vi "StartTrial.vi"(8 "error in (no error)":errorcluster, 11 "TrialBasedExperiment in":refnum<class "OriDiscExperiment.lvclass">) -> (0 "error out":errorcluster, 3 "TrialBasedExperiment out":refnum<class "OriDiscExperiment.lvclass">)   [LabVIEW 2011, in "OriDiscExperiment.lvclass"]
uses:
  OriDiscExperiment.lvclass
  OriDiscExperiment.lvclass/OriDiscExperiment.ctl
  TwoAfcEye/TwoAfcEye.lvclass
panel:
  in  "condRepeatType":string(combo)="None"
  in  "punishType":string(combo)="IncorrRespAndAborts"
  in  "classShown":bool
  in  "classOverride":bool
  in  "correctTargetOnly":bool
  in  "cueTime":dbl
  in  "punishTime":dbl
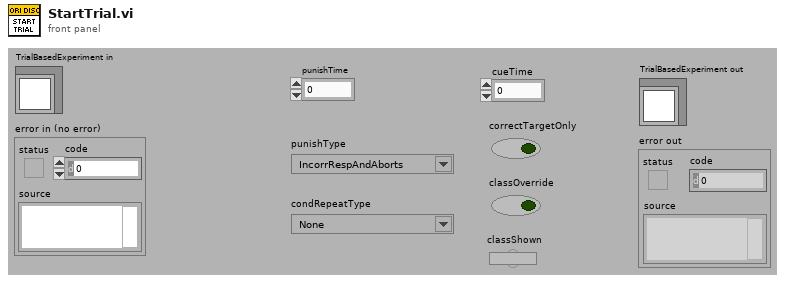
[diagram p1: front panel]
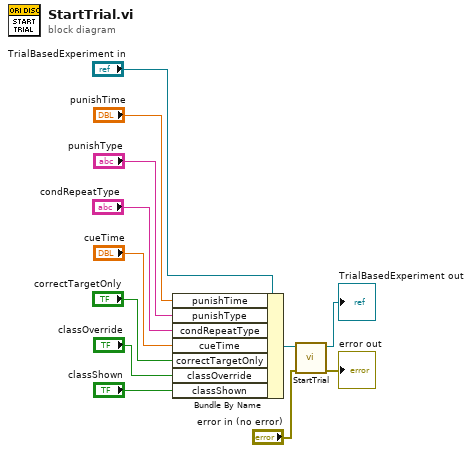
[diagram p0: block diagram]
diagram:
  n1 = Bundle By Name(cluster="TrialBasedExperiment in", "punishTime"="punishTime", "punishType"="punishType", "condRepeatType"="condRepeatType", "cueTime"="cueTime", "correctTargetOnly"="correctTargetOnly", "classOverride"="classOverride", "classShown"="classShown") -> (w5:refnum<class "OriDiscExperiment.lvclass">)
  n2 = call-parent "StartTrial.vi"("error in (no error)"="error in (no error)", "TrialBasedExperiment in"=w5) -> ("error out"=→"error out":errorcluster, "TrialBasedExperiment out"=→"TrialBasedExperiment out":refnum<class "OriDiscExperiment.lvclass">)  [unwired: 8 in]
